vi "Calibrate.vi"(8 "error in (no error)":errorcluster, 11 "34401 in":refnum<class "34401.lvclass">) -> (0 "error out":errorcluster, 1 "Cal Message":string, 2 "Cal Result (Pass=T)":bool, 3 "34401 out":refnum<class "34401.lvclass">)   [LabVIEW 2018, in "34401.lvlib" / "34401.lvclass"]
uses:
  34401.lvclass
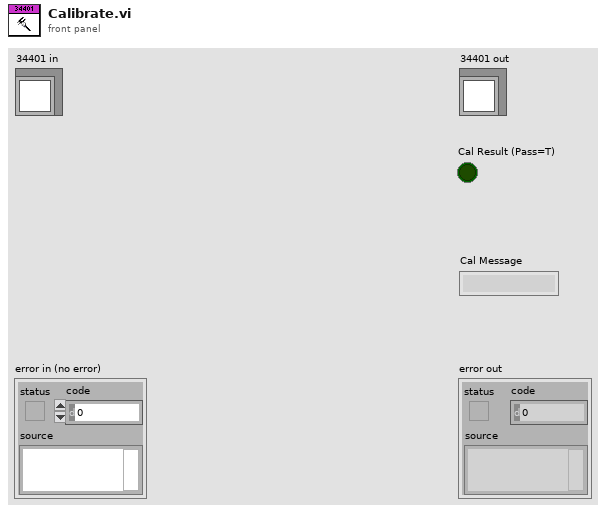
[diagram p1: front panel]
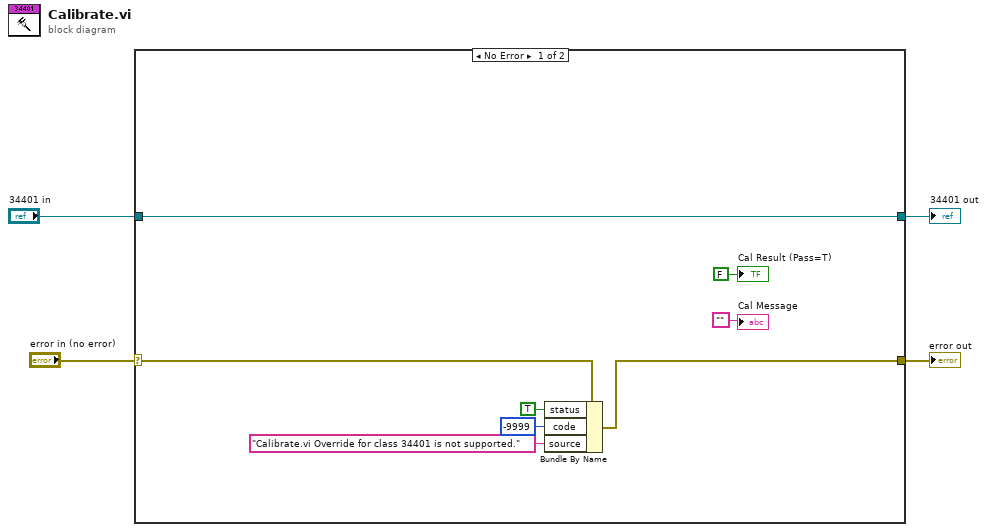
[diagram p0: block diagram]
diagram:
  n1 = case shown="No Error" "error in (no error)" {
    selector: "error in (no error)" -> [w11 w14]
    tunnel: [w10 w14] -> w3
    tunnel: [w12 w13] -> w2
    tunnel: "34401 in" -> [w12 w13]
    frame No Error {
      n2 = Bundle By Name(cluster=w11, "status"=TRUE, "code"=-9999, "source"="Calibrate.vi Override for class 34401 is not supported.") -> (w10:errorcluster)
      "Cal Message" <- ""
      "Cal Result (Pass=T)" <- FALSE ("Cal Result (Pass=T)")
    }
    frame Error {
    }
  }
  "error out" <- w3
  "34401 out" <- w2
